vi "get Komponenten Name.vi"(10 "Gasnummer:":u8, 11 "Array":cluster{"Komponente:":T1, "Konzentration":dbl}[](array[cluster])) -> (3 "String - Ausgabefeld":T2)   [LabVIEW 2020, in "Linearisierung v2.lvlib"]
uses:
  Linearisierung v2.lvlib
  Visualisierungs Elemente/String - Ausgabefeld.ctl
  Visualisierungs Elemente/Auswahlfeld.ctl
  Seiten/FT-IR/FGV FT-IR Gasliste Aktionen.ctl
  Seiten/FT-IR/FT-IR.lvlib
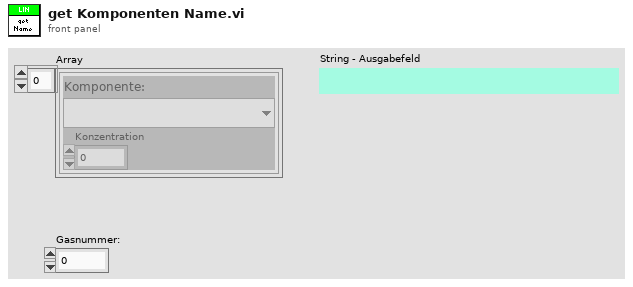
[diagram p1: front panel]
types:
  T1 = typedef "Auswahlfeld.ctl" = u16
  T2 = typedef "String - Ausgabefeld.ctl" = string
  T3 = typedef "FT-IR.lvlib/FGV FT-IR Gasliste Aktionen.ctl" = enum16{"lesen", "Gasliste FT-IR", "Gasliste ausgelesen", "laden", "speichern", "löschen"}
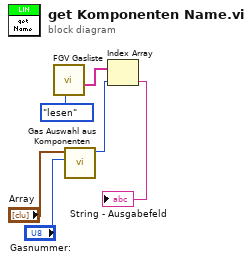
[diagram p0: block diagram]
diagram:
  n1 = call "FGV Gasliste.vi"("Aktionen"=FGV_FT-IR_Gasliste_Aktionen."lesen") -> ("Aktuelle Gasliste gesamt"=w4:T2[])  [unwired: 8 in, 2 out]
  n2 = call "Gas Auswahl aus Komponenten.vi"("Gasnummer:"="Gasnummer:", "Komponentenauswahl"="Array") -> ("Auswahl"=w5:T1)  [unwired: 7 in, 2 out]
  n3 = Index Array(array=w4, index=w5) -> (element=→"String - Ausgabefeld":T2)
